vi "Set Source Value.vi"(8 "error in (no error)":errorcluster, 9 "Source Value Units":T1, 10 "Source Value":dbl, 11 "Power Supply in":refnum<class "Power Supply.lvclass">) -> (0 "error out":errorcluster, 3 "Power Supply out":refnum<class "Power Supply.lvclass">)   [LabVIEW 2011, in "Power Supply.lvclass"]
uses:
  Power Supply.lvclass
  Source Units.ctl
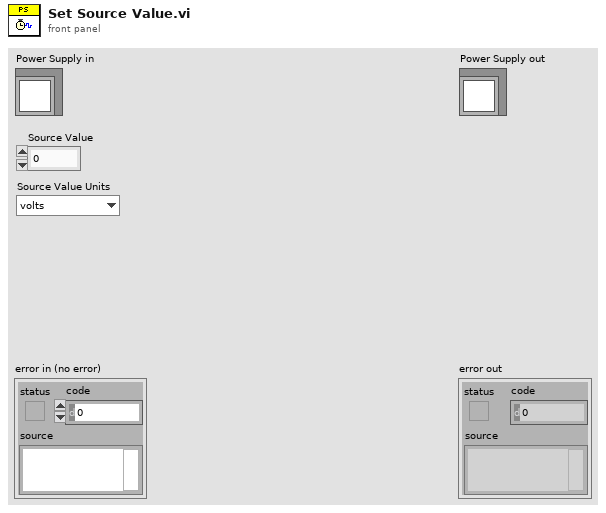
[diagram p1: front panel]
types:
  T1 = typedef "Power Supply.lvclass/Source Units.ctl" = enum16{"volts", "millivolts", "microvolts", "amps", "milliamps", "microamps", "nanoamps"}
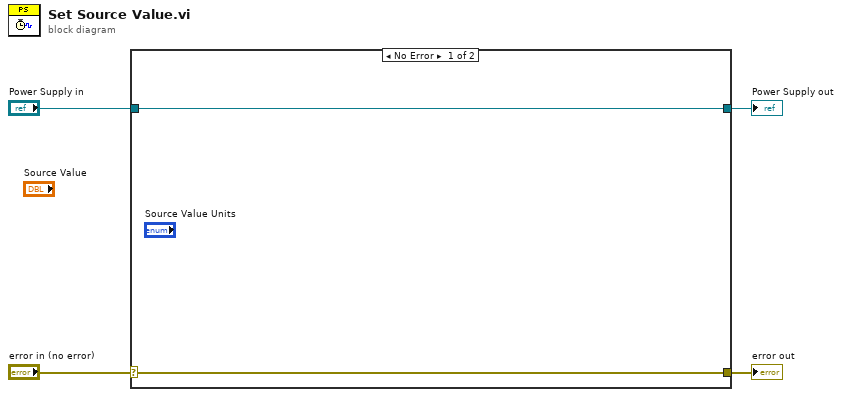
[diagram p0: block diagram]
diagram:
  n1 = case shown="No Error" "error in (no error)" {
    selector: "error in (no error)" -> [w6 w8]
    tunnel: [w6 w8] -> w3
    tunnel: [w5 w7] -> w1
    tunnel: "Power Supply in" -> [w5 w7]
    frame No Error {
    }
    frame Error {
    }
  }
  "error out" <- w3
  "Power Supply out" <- w1
